vi "PAN_SendConnMngr.vi"(6 "timeout in ms (-1)":i32, 9 "connection":T1, 10 "command":string) -> (2 "resp":string)   [LabVIEW 2016]
uses:
  private/vis/PAN_ConnMngrQStruct.ctl
  PAN_TCPSERVER_ConnectionStruct.ctl
panel:
  in  "Cluster":T2
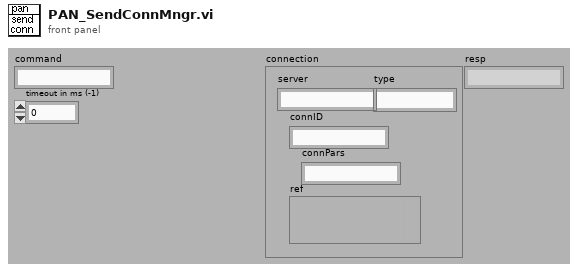
[diagram p1: front panel]
types:
  T1 = typedef "PAN_TCPSERVER_ConnectionStruct.ctl" = cluster{"ref":variant, "connPars":string, "server":string, "connID":string, "type":string}
  T2 = typedef "PAN_ConnMngrQStruct.ctl" = cluster{"action":string, "connection":T1}
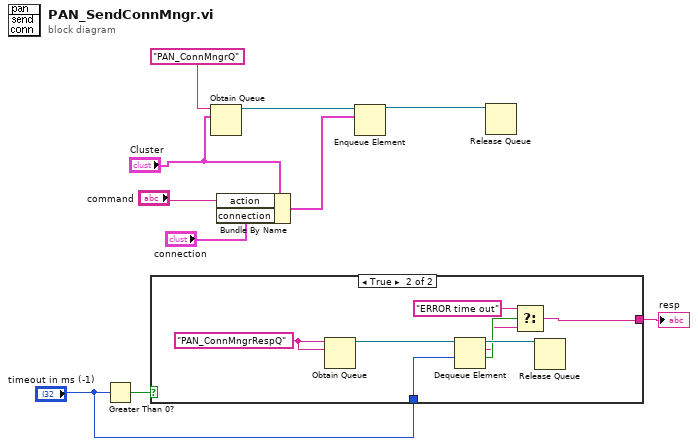
[diagram p0: block diagram]
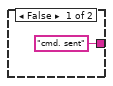
[diagram p2: hidden frame]
diagram:
  n1 = Greater Than 0?(x="timeout in ms (-1)") -> (x > 0?=w2:bool)
  n2 = case shown="True" w2 {
    tunnel: ["cmd. sent" ("name (unnamed)") w13] -> w3
    tunnel: "timeout in ms (-1)" -> [_ w12]
    frame False {
    }
    frame True {
      w19 = "PAN_ConnMngrRespQ" ("name (unnamed)")
      n3 = Obtain Queue(name (unnamed)=w19, element data type=w19) -> (queue out=w18:refnum<queue>)  [unwired: 3 in, 2 out]
      n4 = Dequeue Element(queue=w18, timeout in ms (-1)=w12) -> (queue out=w17:refnum<queue>, element=w15:string, timed out?=w16:bool)  [unwired: 1 in, 1 out]
      n5 = Select(t="ERROR time out", s=w16, f=w15) -> (s? t:f=w13:string)
      n6 = Release Queue(queue=w17) -> ()  [unwired: 1 in, 4 out]
    }
  }
  "resp" <- w3
  n7 = Obtain Queue(name (unnamed)="PAN_ConnMngrQ", element data type="Cluster") -> (queue out=w10:refnum<queue>)  [unwired: 3 in, 2 out]
  n8 = Bundle By Name(cluster="Cluster", "action"="command", "connection"="connection") -> (w8:T2)
  n9 = Enqueue Element(queue=w10, element=w8) -> (queue out=w9:refnum<queue>)  [unwired: 1 in, 3 out]
  n10 = Release Queue(queue=w9) -> ()  [unwired: 1 in, 4 out]
